vi "RandomMoveNumeric.vi"(3 "NumericGameboard":i8[](array[numeric])) -> (1 "Indices":i8[](array[numeric]))   [LabVIEW 2020]
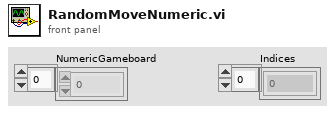
[diagram p1: front panel]
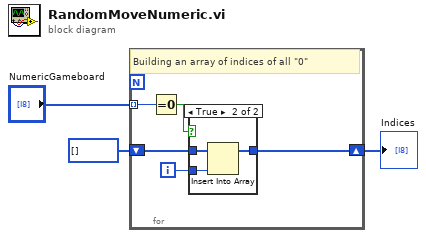
[diagram p0: block diagram]
diagram:
  n1 = for {
    tunnel: "NumericGameboard" -> [w8] mode=indexing
    shift-right: [w5] -> w2
    shift-left: i8[] [] -> [w6]
    i -> [w4]
    # "Building an array of indices of all \"0\""
    n2 = Equal To 0?(x=w8) -> (x = 0?=w7:bool)
    n3 = case shown="True" w7 {
      tunnel: w6 -> [w9 w12]
      tunnel: [w9 w11] -> w5
      tunnel: w4 -> [_ w10]
      frame False {
      }
      frame True {
        n4 = Insert Into Array(array=w12, new element=w10) -> (w11:i8[])  [unwired: 1 in]
      }
    }
  }
  "Indices" <- w2
